vi "scalling parameter.vi"(7 "X":dbl, 8 "E MIN":dbl, 9 "E MAX":dbl, 10 "MIN":dbl, 11 "MAX":dbl) -> (3 "Y":dbl)   [LabVIEW 2018]
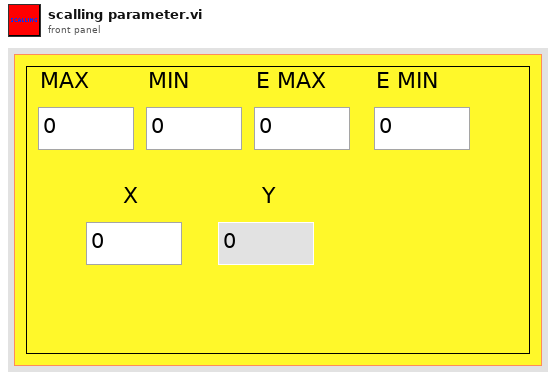
[diagram p1: front panel]
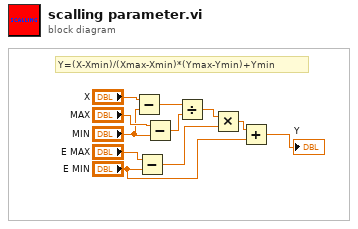
[diagram p0: block diagram]
diagram:
  # "Y=(X-Xmin)/(Xmax-Xmin)*(Ymax-Ymin)+Ymin"
  n1 = Subtract(x="X", y="MIN") -> (x-y=w7:dbl)
  n2 = Subtract(x="E MAX", y="E MIN") -> (x-y=w4:dbl)
  n3 = Subtract(x="MAX", y="MIN") -> (x-y=w6:dbl)
  n4 = Divide(x=w7, y=w6) -> (x/y=w5:dbl)
  n5 = Multiply(x=w5, y=w4) -> (x*y=w3:dbl)
  n6 = Add(x=w3, y="E MIN") -> (x+y=→"Y":dbl)
